vi "return LOX state logic.vi"(0 "system status in":T1={"system state"=enum."Empty & Closed", "fuel level"=0.0, "LOX level"=0.0, "system warnings"={"oxidizer overpress"=FALSE, "oxidizer leak"=FALSE, "fuel overpress"=FALSE, "fuel leak"=FALSE}, "valves"={"fuel load"=FALSE, "fuel return"=FALSE, "fuel comb"=FALSE, "fuel dump"=FALSE, "LOX load"=FALSE, "LOX return"=FALSE, "LOX comb"=FALSE, "LOX dump"=FALSE}, "ignition"=FALSE}, 11 "rocket controls":T4, 12 "LOX over":bool, 13 "LOX leak":bool, 14 "fuel over":bool, 15 "fuel leak":bool) -> (2 "stop loop":bool, 4 "system status out":T1={"system state"=enum."Empty & Closed", "fuel level"=0.0, "LOX level"=0.0, "system warnings"={"oxidizer overpress"=FALSE, "oxidizer leak"=FALSE, "fuel overpress"=FALSE, "fuel leak"=FALSE}, "valves"={"fuel load"=FALSE, "fuel return"=FALSE, "fuel comb"=FALSE, "fuel dump"=FALSE, "LOX load"=FALSE, "LOX return"=FALSE, "LOX comb"=FALSE, "LOX dump"=FALSE}, "ignition"=FALSE})   [LabVIEW 2017]
doc: "This subVI handles the exit logic for the rocket engine simulation LOX loading state.\nIt proceeds to hold when the fuel tank is full or a LOX leak is detected, or to abort when an overpressure is sensed or an abort command is detected.\n\nPaul K Dixon\nP350\nCSUSB"
uses:
  typedefs/user controls.ctl
  typedefs/sysyem status.ctl
  typedefs/system state.ctl
  typedefs/rocket system warnings.ctl
panel:
  # "Standard\nProcedures"
  # "Alternate\nProcedures"
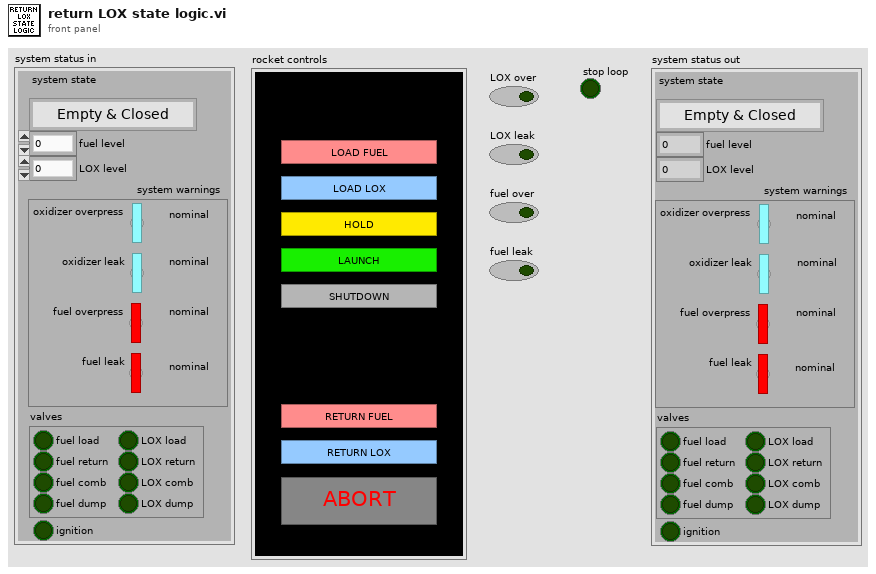
[diagram p1: front panel]
types:
  T1 = typedef "sysyem status.ctl" = cluster{"system state":T2, "fuel level":dbl, "LOX level":dbl, "system warnings":T3, "valves":cluster{"fuel load":bool, "fuel return":bool, "fuel comb":bool, "fuel dump":bool, "LOX load":bool, "LOX return":bool, "LOX comb":bool, "LOX dump":bool}, "ignition":bool}
  T2 = typedef "system state.ctl" = enum16{"Hold", "Empty & Closed", "Launch", "Return Fuel", "Return LOX", "Loading Lox", "Loading Fuel", "Shutdown", "Abort"}
  T3 = typedef "rocket system warnings.ctl" = cluster{"oxidizer overpress":bool, "oxidizer leak":bool, "fuel overpress":bool, "fuel leak":bool}
  T4 = typedef "user controls.ctl" = cluster{"load fuel":bool, "load lox":bool, "hold":bool, "launch":bool, "shutdown":bool, "return fuel":bool, "return lox":bool, "abort":bool}
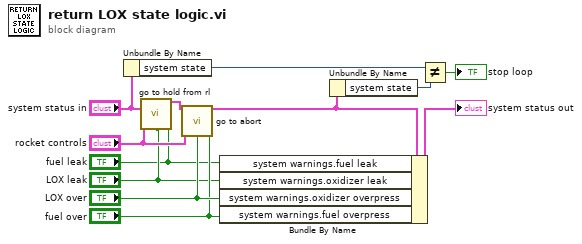
[diagram p0: block diagram]
diagram:
  n1 = Unbundle By Name("system status in") -> ("system state"=w10:T2)
  n2 = call "go to hold from rl.vi"("system status in"="system status in", "rocket controls"="rocket controls", "LOX leak"="LOX leak", "fuel leak"="fuel leak") -> ("system status out"=w1:T1)  [unwired: 11 in]
  n3 = call "go to abort.vi"("system status in"=w1, "rocket controls"="rocket controls", "LOX over"="LOX over", "fuel over"="fuel over") -> ("system status out"=w12:T1)  [unwired: 11 in]
  n4 = Bundle By Name(cluster=w12, "system warnings.fuel leak"="fuel leak", "system warnings.oxidizer leak"="LOX leak", "system warnings.oxidizer overpress"="LOX over", "system warnings.fuel overpress"="fuel over") -> (→"system status out":T1)
  n5 = Unbundle By Name(w12) -> ("system state"=w9:T2)
  n6 = Not Equal?(x=w10, y=w9) -> (x != y?=→"stop loop":bool)
